vi "FC_Get_All_Targets.vi"(7 "Target":T1, 8 "Error In":errorcluster, 11 "Target XML":string) -> (0 "error out":errorcluster, 2 "Array of Targets":string[](array[string]), 3 "Copy of Target XML":string)   [LabVIEW 2014, in "FC_FIRST Client.lvlib"]
doc: "This VI, when given XML data of targets, returns all of the targets contained."
uses:
  FC_FIRST Client.lvlib
  FC_Target.ctl
  <vilib>/regexp/Match Regular Expression.xnode
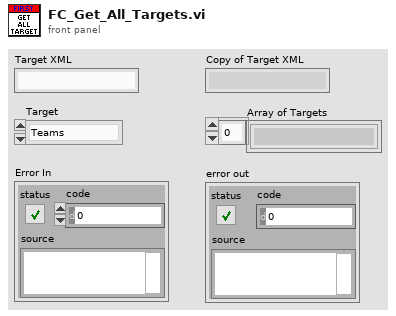
[diagram p1: front panel]
types:
  T1 = typedef "FC_FIRST Client.lvlib/FC_Target.ctl" = enum16{"Teams", "Competitions"}
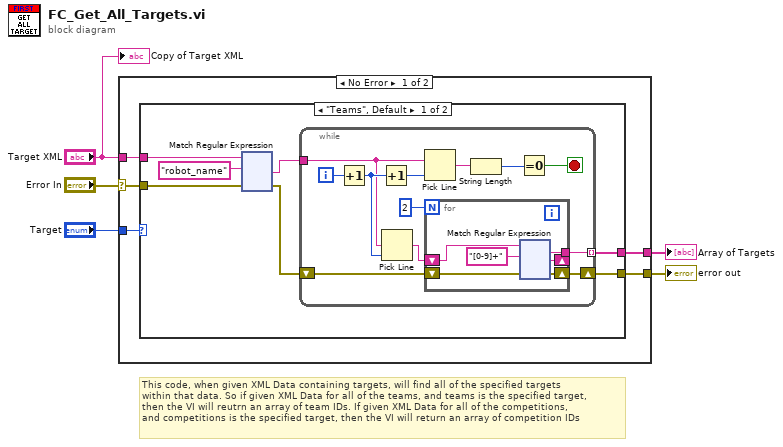
[diagram p0: block diagram]
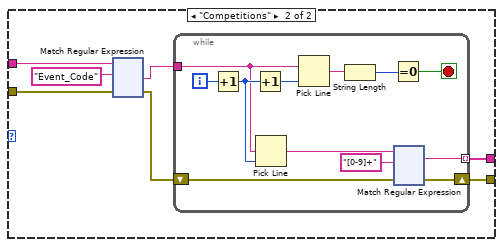
[diagram p2: hidden frame]
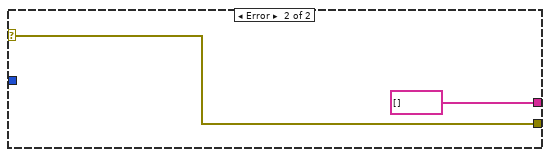
[diagram p3: hidden frame]
diagram:
  # "This code, when given XML Data containing targets, will find all of the specified targets\nwithin that data. So if given XML Data for all of the teams, and teams is the specified target, \nthen the VI will reutrn an array of team IDs. If given XML Data for all of the competitions,\nand competitions is the specified target, then the VI will return an array of competition IDs"
  n1 = case shown="No Error" "Error In" {
    selector: "Error In" -> [w8 w499]
    tunnel: [w10 string[] []] -> w3
    tunnel: [w9 w499] -> w4
    tunnel: "Target XML" -> [w7 _]
    tunnel: "Target" -> [w6 _]
    frame No Error {
      n2 = case shown="\"Teams\", Default" w6 {
        tunnel: [w15 w259] -> w10
        tunnel: [w13 w258] -> w9
        tunnel: w8 -> [w12 w260]
        tunnel: w7 -> [w11 w261]
        frame "Teams", Default {
          n3 = xnode "Match Regular Expression"("input string"=w11, "regular expression"="robot_name", "error in"=w12) -> ("after match"=w16:string, "error out"=w14:errorcluster)  [unwired: 3 in, 3 out]
          n4 = while {
            tunnel: w16 -> [w137]
            tunnel: [w132] -> w15 mode=indexing
            shift-right: [w130] -> w13
            shift-left: w14 -> [w131]
            i -> [w140]
            stop <- w134 stop-if-true
            n5 = Increment(x=w140) -> (x+1=w138:i32)
            n6 = Increment(x=w138) -> (x+1=w139:i32)
            n7 = Pick Line(multi-line string=w137, line index=w138) -> (output string=w129:string)  [unwired: 1 in]
            n8 = Pick Line(multi-line string=w137, line index=w139) -> (output string=w136:string)  [unwired: 1 in]
            n9 = for {
              N: 2 -> [_]
              tunnel: [w145] -> w132
              shift-right: [w143] -> w130
              shift-left: w131 -> [w144]
              shift-right: [w142] -> _
              shift-left: w129 -> [w141]
              n10 = xnode "Match Regular Expression"("input string"=w141, "regular expression"="[0-9]+", "error in"=w144) -> ("whole match"=w145:string, "after match"=w142:string, "error out"=w143:errorcluster)  [unwired: 3 in, 2 out]
            }
            n11 = String Length(string=w136) -> (length=w135:i32)
            n12 = Equal To 0?(x=w135) -> (x = 0?=w134:bool)
          }
        }
        frame "Competitions" {
          n13 = xnode "Match Regular Expression"("input string"=w261, "regular expression"="Event_Code", "error in"=w260) -> ("after match"=w263:string, "error out"=w262:errorcluster)  [unwired: 3 in, 3 out]
          n14 = while {
            tunnel: w263 -> [w384]
            tunnel: [w379] -> w259 mode=indexing
            shift-right: [w377] -> w258
            shift-left: w262 -> [w378]
            i -> [w387]
            stop <- w381 stop-if-true
            n15 = Increment(x=w387) -> (x+1=w385:i32)
            n16 = Increment(x=w385) -> (x+1=w386:i32)
            n17 = Pick Line(multi-line string=w384, line index=w385) -> (output string=w380:string)  [unwired: 1 in]
            n18 = Pick Line(multi-line string=w384, line index=w386) -> (output string=w383:string)  [unwired: 1 in]
            n19 = String Length(string=w383) -> (length=w382:i32)
            n20 = Equal To 0?(x=w382) -> (x = 0?=w381:bool)
            n21 = xnode "Match Regular Expression"("input string"=w380, "regular expression"="[0-9]+", "error in"=w378) -> ("whole match"=w379:string, "error out"=w377:errorcluster)  [unwired: 3 in, 3 out]
          }
        }
      }
    }
    frame Error {
    }
  }
  "Array of Targets" <- w3
  "error out" <- w4
  "Copy of Target XML" <- "Target XML"
